vi "Prune.vi"(8 "error in (no error)":errorcluster, 10 "Master Device in":refnum<class "Master Device.lvclass">, 11 "Master Device in":refnum<class "Master Device.lvclass">) -> (0 "error out":errorcluster, 2 "Master Device out":refnum<class "Master Device.lvclass">, 3 "Master Device out":refnum<class "Master Device.lvclass">)   [LabVIEW 2013, in "Master Device.lvclass"]
doc: "Required by Device for override, the Master Device only includes this as a \"stub.\" See override of FinalizeHWI for master code (or specific child of master)."
uses:
  Master Device.lvclass
  Device/Device.lvclass
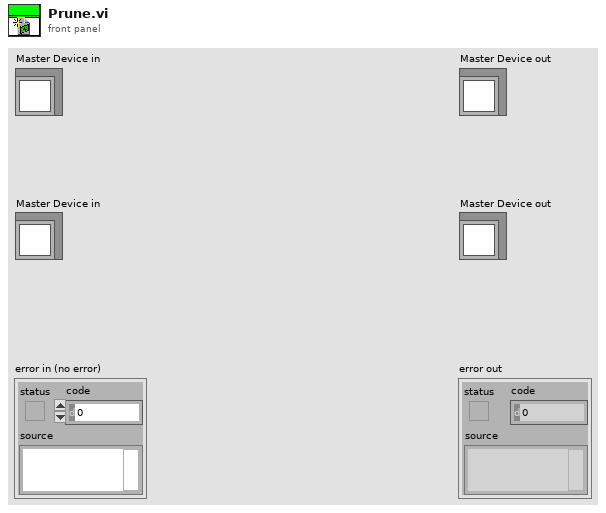
[diagram p1: front panel]
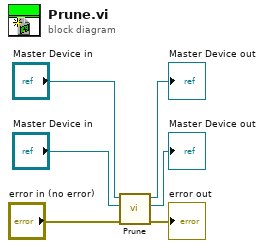
[diagram p0: block diagram]
diagram:
  n1 = call-parent "Prune.vi"("error in (no error)"="error in (no error)", "Master Device in"="Master Device in", "Device in"="Master Device in") -> ("error out"=→"error out":errorcluster, "Master Device out"=→"Master Device out":refnum<class "Master Device.lvclass">, "Device out"=→"Master Device out":refnum<class "Master Device.lvclass">)  [unwired: 6 in]
